vi "Gas_management_global.vi"() -> ()   [LabVIEW 2010]
panel:
  in  "Hi Tec Calib names":string[](array[string])
  in  "Hi Tec Calibrations":dbl[][](array[numeric]) format="%.2f"
  out "Gas Control Client":string
  out "Carrier 2 Gas":string
  out "Carrier 1 Gas":string
  out "Trace Gas":string
  out "Carrier 1 Hi-Tec Range":string
  out "Trace Hi-Tec Range":string
  in  "Atmos Pres (mbars)":dbl=1000.0 format="%.2f"
  in  "Release temp (deg C)":dbl=20.0 format="%.2f"
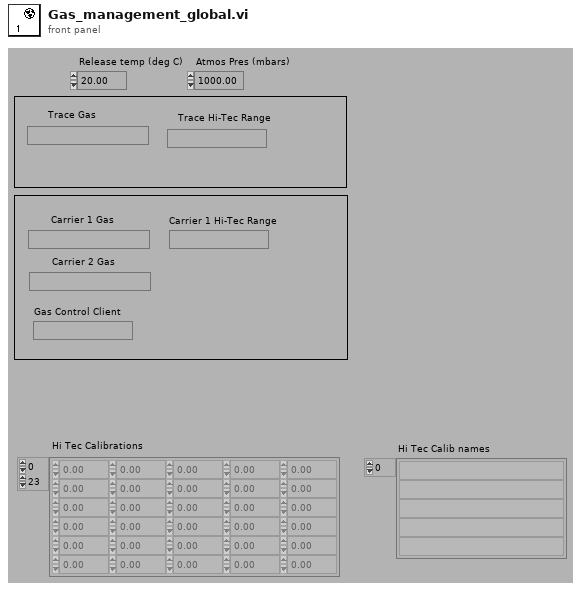
[diagram p1: front panel]
diagram:
